vi "CRYNext Freq.vi"(3 "No. Steps":i32=1, 4 "Freq In":dbl=100.0 format="%.2f", 5 "Step size":u16(ring) items=["R10 (1/3 Oct.)", "R20 (1/6 Oct.)", "R40 (1/12 Oct.)", "R80 (1/24 Oct.)", "1/1 Octave"]) -> (2 "Next Freq":dbl=125.0 format="%.2f")   [LabVIEW 2013]
uses:
  CRYStimulus Global.vi
panel:
  # "This VI finds the next frequency\nto the input frequency in the chosen series."
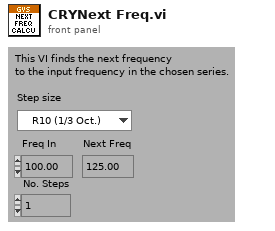
[diagram p1: front panel]
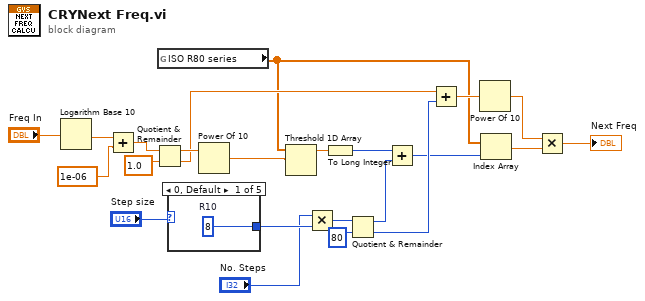
[diagram p0: block diagram]
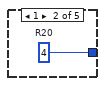
[diagram p2: hidden frame]
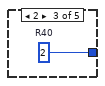
[diagram p3: hidden frame]
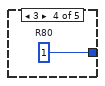
[diagram p4: hidden frame]
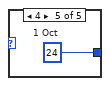
[diagram p5: hidden frame]
diagram:
  n1 = Logarithm Base 10(1:"Freq In") -> (0:w12:dbl)
  n2 = Add(x=w12, y=1e-06) -> (x+y=w10:dbl)
  n3 = Quotient & Remainder(x=w10, y=1.0) -> (x-y*floor(x/y)=w18:dbl, floor(x/y)=w6:dbl)
  n4 = global read "CRYStimulus Global.vi" "ISO R80 series"() -> (w1:dbl[])
  n5 = case shown="0, Default" "Step size" {
    tunnel: [w24 w25 w26 w27 w28] -> w22
    frame 0, Default {
      w24 = 8  # R10
    }
    frame 1 {
      w25 = 4  # R20
    }
    frame 2 {
      w26 = 2  # R40
    }
    frame 3 {
      w27 = 1  # R80
    }
    frame 4 {
      w28 = 24  # 1 Oct
    }
  }
  n6 = Power Of 10(x=w18) -> (10^x=w17:dbl)
  n7 = Threshold 1D Array(2:w17, 3:w1) -> (0:w21:dbl)  [unwired: 1 out]
  n8 = Multiply(x="No. Steps", y=w22) -> (x*y=w7:i32)
  n9 = To Long Integer(number=w21) -> (32bit integer=w20:i32)
  n10 = Quotient & Remainder(x=w7, y=80 ("No. Steps")) -> (x-y*floor(x/y)=w3:i32, floor(x/y)=w5:i32)
  n11 = Add(x=w20, y=w3) -> (x+y=w2:i32)
  n12 = Add(x=w6, y=w5) -> (x+y=w4:dbl)
  n13 = Power Of 10(x=w4) -> (10^x=w13:dbl)
  n14 = Index Array(array=w1, index=w2) -> (element=w16:dbl)
  n15 = Multiply(x=w13, y=w16) -> (x*y=→"Next Freq":dbl)
